vi "Table Prefix.vi"() -> (0 "DB Table Prefix":string)   [LabVIEW 2012, in "DB-Configuration.lvlib"]
doc: "Prefix for configuration tables created in Oracle.\n\nEdit the prefix constant to your needs."
uses:
  DB-Configuration.lvlib
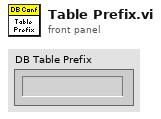
[diagram p1: front panel]
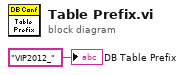
[diagram p0: block diagram]
diagram:
  "DB Table Prefix" <- "VIP2012_" ("DB Table Prefix")
